vi "Electrode to Color.vi"(1 "Electrode Type":string) -> (0 "Color":u32)   [LabVIEW 2020, in "Retrieve and Visualize.lvclass"]
uses:
  Retrieve and Visualize.lvclass
  Retrieve and Visualize.lvclass/Retrieve and Visualize.ctl
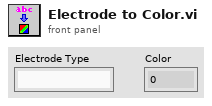
[diagram p1: front panel]
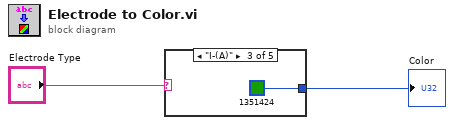
[diagram p0: block diagram]
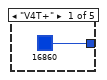
[diagram p2: hidden frame]
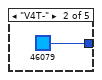
[diagram p3: hidden frame]
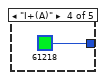
[diagram p4: hidden frame]
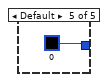
[diagram p5: hidden frame]
diagram:
  n1 = case shown="\"I-(A)\"" "Electrode Type" {
    tunnel: [u32 16860 u32 46079 u32 1351424 u32 61218 u32 0] -> w2
    frame "V4T+" {
    }
    frame "V4T-" {
    }
    frame "I-(A)" {
    }
    frame "I+(A)" {
    }
    frame Default {
    }
  }
  "Color" <- w2
